vi "Write_flag-state.vi"(8 "error in (no error)":errorcluster, 10 "flag state":bool, 11 "flag in":refnum<class "flag.lvclass">) -> (0 "error out":errorcluster, 3 "flag out":refnum<class "flag.lvclass">)   [LabVIEW 2017, in "flag.lvclass"]
uses:
  flag.lvclass
  flag.lvclass/flag.ctl
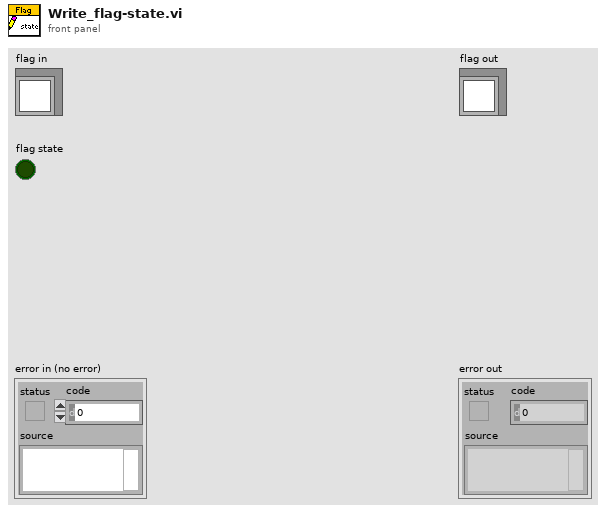
[diagram p1: front panel]
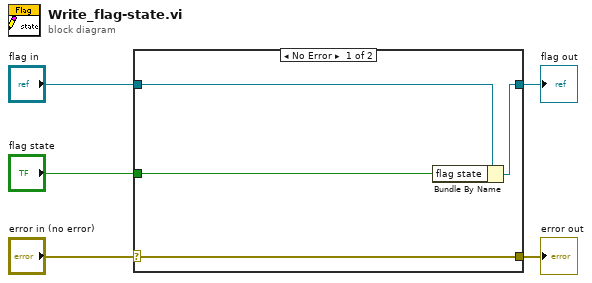
[diagram p0: block diagram]
diagram:
  n1 = case shown="No Error" "error in (no error)" {
    selector: "error in (no error)" -> [w9 w10]
    tunnel: [w9 w10] -> w4
    tunnel: [w7 w11] -> w2
    tunnel: "flag in" -> [w8 w11]
    tunnel: "flag state" -> [w6 _]
    frame No Error {
      n2 = Bundle By Name(cluster=w8, "flag state"=w6) -> (w7:refnum<class "flag.lvclass">)
    }
    frame Error {
    }
  }
  "error out" <- w4
  "flag out" <- w2
